vi "Read Speed Schedule.vi"(8 "error in (no error)":errorcluster, 11 "ObjectSettings in":refnum<class "ObjectSettings.lvclass">) -> (0 "error out":errorcluster, 2 "Schedule":u16(ring) items=["Constant", "Ramp", "Function", "Formula"], 3 "ObjectSettings out":refnum<class "ObjectSettings.lvclass">)   [LabVIEW 2019, in "ObjectSettings.lvclass"]
uses:
  ObjectSettings.lvclass
  ObjectSettings.lvclass/ObjectSettings.ctl
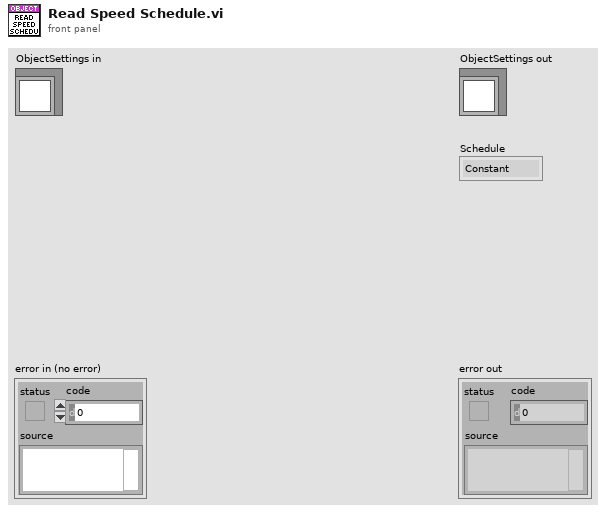
[diagram p1: front panel]
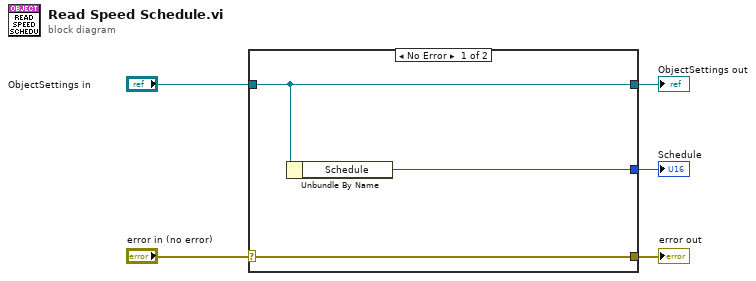
[diagram p0: block diagram]
diagram:
  n1 = case shown="No Error" "error in (no error)" {
    selector: "error in (no error)" -> [w8 w9]
    tunnel: [w8 w9] -> w4
    tunnel: [w7 w10] -> w2
    tunnel: "ObjectSettings in" -> [w7 w10]
    tunnel: [w6 _] -> w1
    frame No Error {
      n2 = Unbundle By Name(w7) -> ("Schedule"=w6:u16)
    }
    frame Error {
    }
  }
  "error out" <- w4
  "ObjectSettings out" <- w2
  "Schedule" <- w1
